vi "VariantToCluster.vi"(8 "error in (no error)":errorcluster, 11 "Cluster":variant) -> (0 "error out":errorcluster, 1 "cluster elements info":variant[](array[variant]), 2 "Cluster element names":string[](array[string]), 3 "Cluster elements":variant[](array[variant]))   [LabVIEW 2019, in "BlueVariantView.lvlib"]
uses:
  BlueVariantView.lvlib
  <vilib>/Utility/Data Type/NI_Data Type.lvlib
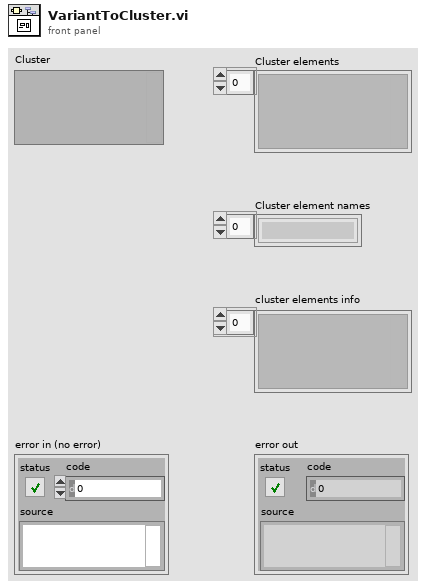
[diagram p1: front panel]
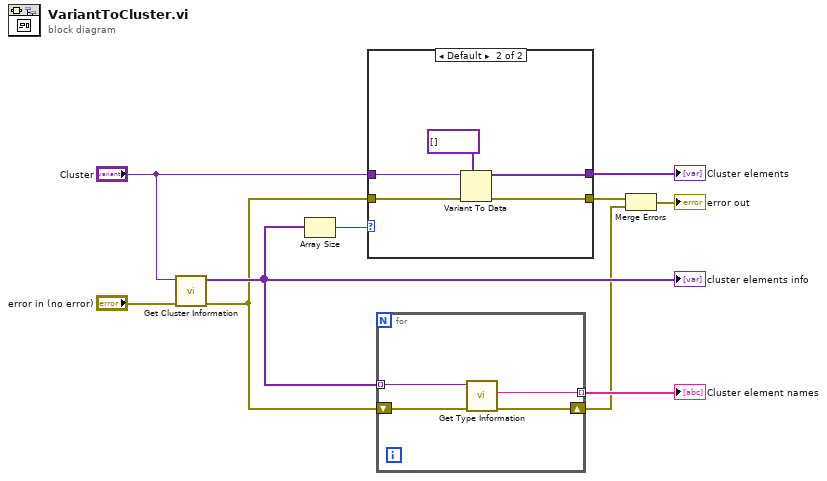
[diagram p0: block diagram]
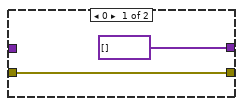
[diagram p2: hidden frame]
diagram:
  n1 = call <vilib>:"Get Cluster Information.vi"("error in (no error)"="error in (no error)", "variant"="Cluster") -> ("error out"=w4:errorcluster, "cluster elements"=w6:variant[])  [unwired: 8 in]
  "cluster elements info" <- w6
  n2 = Array Size(array=w6) -> (size(s)=w8:i32)
  n3 = case shown="Default" w8 {
    tunnel: "Cluster" -> [_ w16]
    tunnel: w4 -> [w11 w15]
    tunnel: [variant[] [] w14] -> w7
    tunnel: [w11 w13] -> w3
    frame 0 {
    }
    frame Default {
      n4 = Variant To Data(error in=w15, type=variant[] [], Variant=w16) -> (data=w14:variant[], error out=w13:errorcluster)
    }
  }
  "Cluster elements" <- w7
  n5 = for {
    tunnel: w6 -> [w21] mode=indexing
    tunnel: [w20] -> w5 mode=indexing
    shift-right: [w18] -> w2
    shift-left: w4 -> [w19]
    n6 = call <vilib>:"Get Type Information.vi"("error in (no error)"=w19, "variant"=w21) -> ("error out"=w18:errorcluster, "name"=w20:string)  [unwired: 5 in, 3 out]
  }
  "Cluster element names" <- w5
  n7 = Merge Errors(w3, w2) -> (→"error out":errorcluster)
